vi "TcA02-005_ResizingAttributesCanBeModifiedFasterThanGOOP1.vi"(1 "Input buffer":T3="1", 3 "Invocation info":T2, 5 "error in (no error)":errorcluster, 6 "Add log to result?":bool) -> (16 "Test Data":T1 {"Numeric Measurement" format="%.2f"}, 19 "error out":errorcluster)   [LabVIEW 2020]
doc: "Test case template."
uses:
  Shared/Support_InputBuffer.ctl
  Shared/Support_InvocationInfo.ctl
  Shared/Support_TestData.ctl
  Shared/Support_ResultType.ctl
  TestClasses/G#SubClass1_class/G#SubClass1.lvclass
  TestClasses/G#BaseClass1_class/G#BaseClass1.lvclass
  <vilib>/addons/_AddQ/G#Object/G#Object.lvclass
panel:
  in  "Test name":string="TcA02-005 Resizing attributes can be modified faster than GOOP1"
  out "Test result":bool
  out "Result":string
  # "Verify that object attributes are modified faster\nthan GOOP1 for an attribute that resizes."
  # "Sub test case"
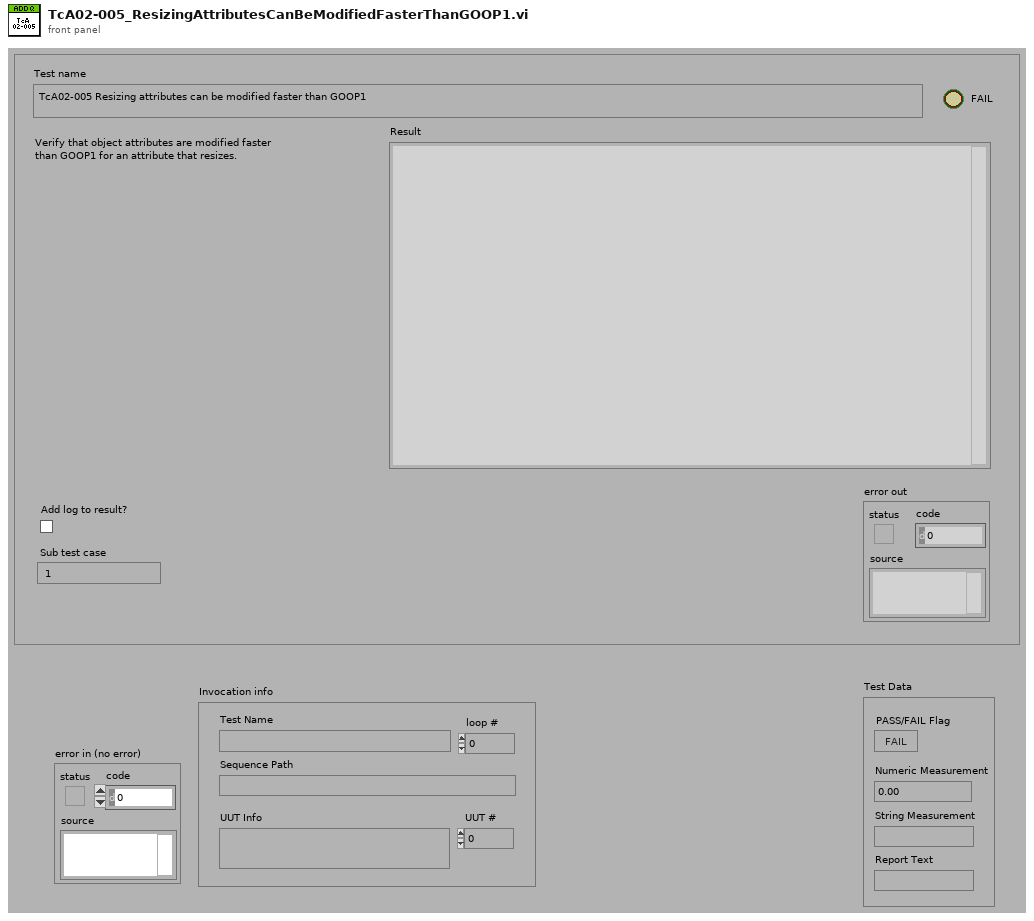
[diagram p1: front panel]
types:
  T1 = typedef "Support_TestData.ctl" = cluster{"PASS/FAIL Flag":bool, "Numeric Measurement":dbl, "String Measurement":string, "Report Text":string}
  T2 = typedef "Support_InvocationInfo.ctl" = cluster{"UUT #":i32, "loop #":i32, "UUT Info":string, "Test Name":string, "Sequence Path":path}
  T3 = typedef "Support_InputBuffer.ctl" = string
  T4 = typedef "Support_ResultType.ctl" = cluster{"Pass":bool, "Comment":string, "MeasurementValue":dbl}
  T5 = typedef "TcOldClass_Object Reference.ctl" = refnum<k1>
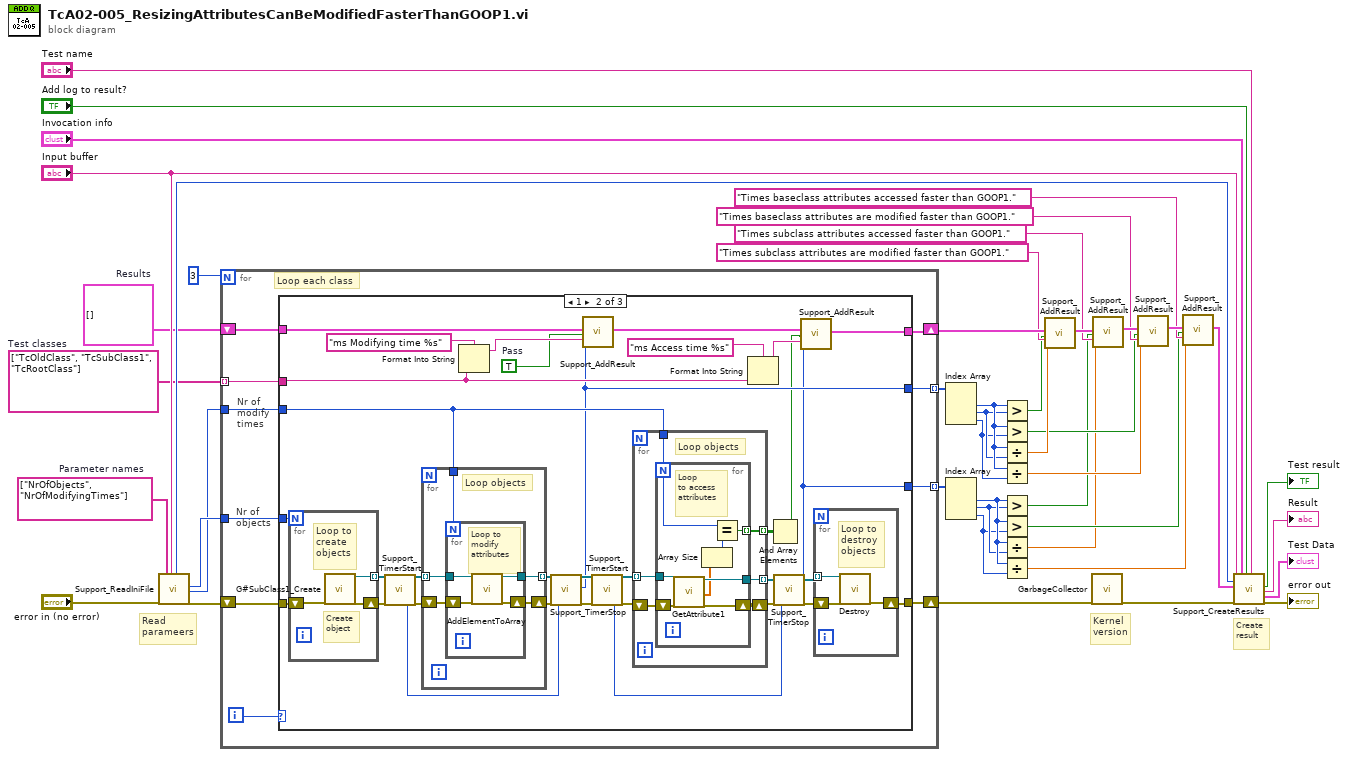
[diagram p0: block diagram]
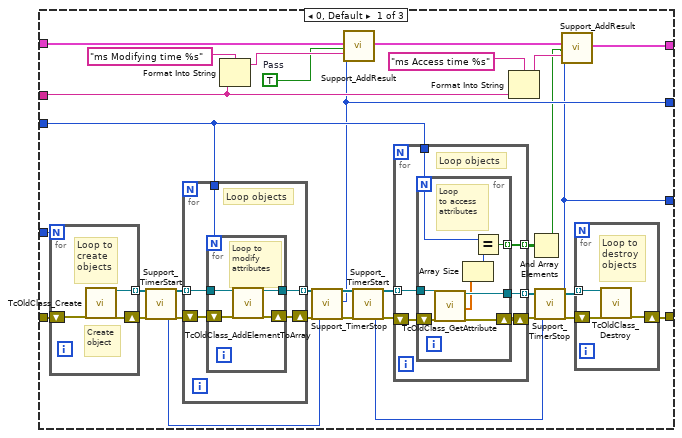
[diagram p2: hidden frame]
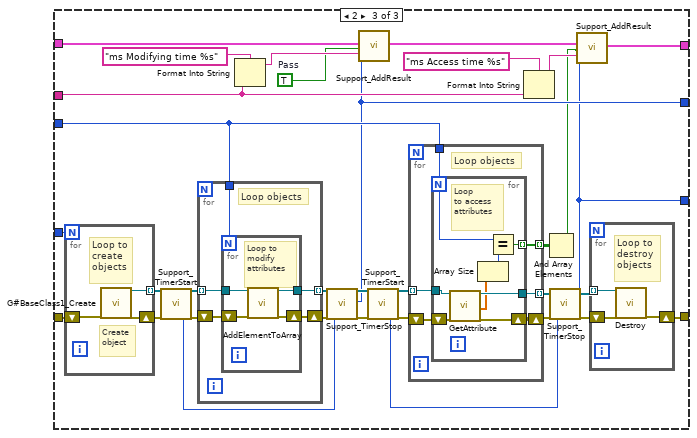
[diagram p3: hidden frame]
diagram:
  w26 = string[] ["TcOldClass", "TcSubClass1", "TcRootClass"]  # Test classes
  w27 = T4[] []  # Results
  w29 = string[] ["NrOfObjects", "NrOfModifyingTimes"]  # Parameter names
  # "Kernel\nversion"
  # "Read\nparameers"
  # "Create\nresult"
  n1 = call "Support_ReadIniFile.vi"("error in (no error)"="error in (no error)", "Parameter names"=w29, "Sub test case"="Input buffer") -> ("Timer start"=w34:u32, "Parameter1 as I32"=w30:i32, "Parameter2 as I32"=w28:i32, "error out"=w31:errorcluster)  [unwired: 9 in, 4 out]
  n2 = for {
    N: 3 -> [_]
    tunnel: w30 -> [w54]
    shift-right: [w52] -> w32
    shift-left: w31 -> [w51]
    tunnel: w28 -> [w50]
    shift-right: [w47] -> w24
    shift-left: w27 -> [w48]
    tunnel: w26 -> [w49] mode=indexing
    tunnel: [w46] -> w20 mode=indexing
    tunnel: [w45] -> w21 mode=indexing
    i -> [w53]
    # "Nr of\nobjects"
    # "Nr of\nmodify\ntimes"
    # "Loop each class"
    n3 = case shown="1" w53 {
      tunnel: w51 -> [w81 w139 w197]
      tunnel: w54 -> [w83 w141 w199]
      tunnel: [w73 w131 w189] -> w52
      tunnel: w50 -> [w70 w128 w186]
      tunnel: w49 -> [w61 w119 w177]
      tunnel: w48 -> [w67 w125 w183]
      tunnel: [w60 w118 w176] -> w47
      tunnel: [w59 w117 w175] -> w46
      tunnel: [w58 w116 w174] -> w45
      frame 0, Default {
        w57 = TRUE  # Pass
        n4 = for {
          N: w83 -> [_]
          shift-right: [w110] -> w80
          shift-left: w81 -> [w111]
          tunnel: [w112] -> w79 mode=indexing
          # "Create\nobject"
          # "Loop to\ncreate\nobjects"
          n5 = call "TcOldClass_Create.vi"("error in (no error)"=w111) -> ("reference"=w112:T5, "error out"=w110:errorcluster)  [unwired: 17 in]
        }
        n6 = call "Support_TimerStart.vi"("error in (no error)"=w80) -> ("Start time"=w82:u32, "error out"=w78:errorcluster)  [unwired: 17 in]
        n7 = for {
          tunnel: w79 -> [w88] mode=indexing
          tunnel: w70 -> [w87]
          tunnel: [w86] -> w71 mode=indexing
          shift-right: [w84] -> w77
          shift-left: w78 -> [w85]
          # "Loop objects"
          n8 = for {
            N: w87 -> [_]
            shift-right: [w91] -> w84
            shift-left: w85 -> [w92]
            tunnel: w88 -> [w90]
            tunnel: [w89] -> w86
            # "Loop to\nmodify\nattributes"
            n9 = call "TcOldClass_AddElementToArray.vi"("reference"=w90, "error in (no error)"=w92) -> ("duplicate reference"=w89:T5, "error out"=w91:errorcluster)  [unwired: 16 in]
          }
        }
        n10 = Format Into String(format string="ms Modifying time %s", w61) -> (resulting string=w65:string)  [unwired: 2 in, 1 out]
        n11 = call "Support_TimerStop.vi"("error in (no error)"=w77, "Start time"=w82) -> ("Time (ms)"=w59:u32, "error out"=w76:errorcluster)  [unwired: 16 in]
        n12 = call "Support_AddResult.vi"("Results in"=w67, "Pass"=w57, "Comment"=w65, "MeasurementValue"=w59) -> ("Results out"=w64:T4[])  [unwired: 15 in]
        n13 = call "Support_TimerStart.vi"("error in (no error)"=w76) -> ("Start time"=w68:u32, "error out"=w75:errorcluster)  [unwired: 17 in]
        n14 = for {
          shift-right: [w97] -> w74
          shift-left: w75 -> [w98]
          tunnel: w71 -> [w96] mode=indexing
          tunnel: w70 -> [w95]
          tunnel: [w94] -> w69 mode=indexing
          tunnel: [w93] -> w55 mode=indexing
          # "Loop objects"
          n15 = for {
            N: w95 -> [w100]
            shift-right: [w105] -> w97
            shift-left: w98 -> [w106]
            tunnel: w96 -> [w104]
            tunnel: [w103] -> w94
            tunnel: [w99] -> w93 mode=indexing
            # "Loop\nto access\nattributes"
            n16 = call "TcOldClass_GetAttribute.vi"("reference"=w104, "error in (no error)"=w106) -> ("duplicate reference"=w103:T5, "tcRootArray"=w102:dbl[], "error out"=w105:errorcluster)  [unwired: 13 in, 2 out]
            n17 = Array Size(array=w102) -> (size(s)=w101:i32)
            n18 = Equal?(x=w100, y=w101) -> (x = y?=w99:bool)
          }
        }
        n19 = Format Into String(format string="ms Access time %s", w61) -> (resulting string=w63:string)  [unwired: 2 in, 1 out]
        n20 = And Array Elements(Boolean array=w55) -> (logical AND=w56:bool)
        n21 = call "Support_TimerStop.vi"("error in (no error)"=w74, "Start time"=w68) -> ("Time (ms)"=w58:u32, "error out"=w72:errorcluster)  [unwired: 16 in]
        n22 = call "Support_AddResult.vi"("Results in"=w64, "Pass"=w56, "Comment"=w63, "MeasurementValue"=w58) -> ("Results out"=w60:T4[])  [unwired: 15 in]
        n23 = for {
          tunnel: w69 -> [w109] mode=indexing
          shift-right: [w107] -> w73
          shift-left: w72 -> [w108]
          # "Loop to \ndestroy\nobjects"
          n24 = call "TcOldClass_Destroy.vi"("reference"=w109, "error in (no error)"=w108) -> ("error out"=w107:errorcluster)  [unwired: 17 in]
        }
      }
      frame 1 {
        w115 = TRUE  # Pass
        n25 = for {
          N: w141 -> [_]
          shift-right: [w169] -> w138
          shift-left: w139 -> [w170]
          tunnel: [w168] -> w137 mode=indexing
          # "Create\nobject"
          # "Loop to\ncreate\nobjects"
          n26 = call "G#SubClass1_Create.vi"("error in (no error)"=w170) -> ("reference out"=w168:refnum<class "G#SubClass1.lvclass">, "error out"=w169:errorcluster)  [unwired: 16 in, 1 out]
        }
        n27 = call "Support_TimerStart.vi"("error in (no error)"=w138) -> ("Start time"=w140:u32, "error out"=w136:errorcluster)  [unwired: 17 in]
        n28 = for {
          tunnel: w137 -> [w146] mode=indexing
          tunnel: w128 -> [w145]
          tunnel: [w144] -> w129 mode=indexing
          shift-right: [w142] -> w135
          shift-left: w136 -> [w143]
          # "Loop objects"
          n29 = for {
            N: w145 -> [_]
            shift-right: [w149] -> w142
            shift-left: w143 -> [w150]
            tunnel: w146 -> [w148]
            tunnel: [w147] -> w144
            # "Loop to\nmodify\nattributes"
            n30 = call-dynamic "AddElementToArray.vi"("reference in"=w148, "error in (no error)"=w150) -> ("reference out"=w147:refnum<class "G#SubClass1.lvclass">, "error out"=w149:errorcluster)  [unwired: 16 in]
          }
        }
        n31 = Format Into String(format string="ms Modifying time %s", w119) -> (resulting string=w123:string)  [unwired: 2 in, 1 out]
        n32 = call "Support_TimerStop.vi"("error in (no error)"=w135, "Start time"=w140) -> ("Time (ms)"=w117:u32, "error out"=w134:errorcluster)  [unwired: 16 in]
        n33 = call "Support_AddResult.vi"("Results in"=w125, "Pass"=w115, "Comment"=w123, "MeasurementValue"=w117) -> ("Results out"=w122:T4[])  [unwired: 15 in]
        n34 = call "Support_TimerStart.vi"("error in (no error)"=w134) -> ("Start time"=w126:u32, "error out"=w133:errorcluster)  [unwired: 17 in]
        n35 = for {
          shift-right: [w155] -> w132
          shift-left: w133 -> [w156]
          tunnel: w129 -> [w154] mode=indexing
          tunnel: w128 -> [w153]
          tunnel: [w152] -> w127 mode=indexing
          tunnel: [w151] -> w113 mode=indexing
          # "Loop objects"
          n36 = for {
            N: w153 -> [w158]
            shift-right: [w163] -> w155
            shift-left: w156 -> [w164]
            tunnel: w154 -> [w162]
            tunnel: [w161] -> w152
            tunnel: [w157] -> w151 mode=indexing
            # "Loop\nto access\nattributes"
            n37 = call-dynamic "GetAttribute1.vi"("reference in"=w162, "error in (no error)"=w164) -> ("reference out"=w161:refnum<class "G#SubClass1.lvclass">, "Base class.Array"=w160:dbl[], "error out"=w163:errorcluster)  [unwired: 13 in, 2 out]
            n38 = Array Size(array=w160) -> (size(s)=w159:i32)
            n39 = Equal?(x=w158, y=w159) -> (x = y?=w157:bool)
          }
        }
        n40 = Format Into String(format string="ms Access time %s", w119) -> (resulting string=w121:string)  [unwired: 2 in, 1 out]
        n41 = And Array Elements(Boolean array=w113) -> (logical AND=w114:bool)
        n42 = call "Support_TimerStop.vi"("error in (no error)"=w132, "Start time"=w126) -> ("Time (ms)"=w116:u32, "error out"=w130:errorcluster)  [unwired: 16 in]
        n43 = call "Support_AddResult.vi"("Results in"=w122, "Pass"=w114, "Comment"=w121, "MeasurementValue"=w116) -> ("Results out"=w118:T4[])  [unwired: 15 in]
        n44 = for {
          tunnel: w127 -> [w167] mode=indexing
          shift-right: [w165] -> w131
          shift-left: w130 -> [w166]
          # "Loop to \ndestroy\nobjects"
          n45 = call-dynamic "Destroy.vi"("reference in"=w167, "error in (no error)"=w166) -> ("error out"=w165:errorcluster)  [unwired: 16 in, 1 out]
        }
      }
      frame 2 {
        w173 = TRUE  # Pass
        n46 = for {
          N: w199 -> [_]
          shift-right: [w227] -> w196
          shift-left: w197 -> [w228]
          tunnel: [w226] -> w195 mode=indexing
          # "Create\nobject"
          # "Loop to\ncreate\nobjects"
          n47 = call "G#BaseClass1_Create.vi"("error in (no error)"=w228) -> ("reference out"=w226:refnum<class "G#BaseClass1.lvclass">, "error out"=w227:errorcluster)  [unwired: 16 in, 1 out]
        }
        n48 = call "Support_TimerStart.vi"("error in (no error)"=w196) -> ("Start time"=w198:u32, "error out"=w194:errorcluster)  [unwired: 17 in]
        n49 = for {
          tunnel: w195 -> [w204] mode=indexing
          tunnel: w186 -> [w203]
          tunnel: [w202] -> w187 mode=indexing
          shift-right: [w200] -> w193
          shift-left: w194 -> [w201]
          # "Loop objects"
          n50 = for {
            N: w203 -> [_]
            shift-right: [w207] -> w200
            shift-left: w201 -> [w208]
            tunnel: w204 -> [w206]
            tunnel: [w205] -> w202
            # "Loop to\nmodify\nattributes"
            n51 = call-dynamic "AddElementToArray.vi"("reference in"=w206, "error in (no error)"=w208) -> ("reference out"=w205:refnum<class "G#BaseClass1.lvclass">, "error out"=w207:errorcluster)  [unwired: 16 in]
          }
        }
        n52 = Format Into String(format string="ms Modifying time %s", w177) -> (resulting string=w181:string)  [unwired: 2 in, 1 out]
        n53 = call "Support_TimerStop.vi"("error in (no error)"=w193, "Start time"=w198) -> ("Time (ms)"=w175:u32, "error out"=w192:errorcluster)  [unwired: 16 in]
        n54 = call "Support_AddResult.vi"("Results in"=w183, "Pass"=w173, "Comment"=w181, "MeasurementValue"=w175) -> ("Results out"=w180:T4[])  [unwired: 15 in]
        n55 = call "Support_TimerStart.vi"("error in (no error)"=w192) -> ("Start time"=w184:u32, "error out"=w191:errorcluster)  [unwired: 17 in]
        n56 = for {
          shift-right: [w213] -> w190
          shift-left: w191 -> [w214]
          tunnel: w187 -> [w212] mode=indexing
          tunnel: w186 -> [w211]
          tunnel: [w210] -> w185 mode=indexing
          tunnel: [w209] -> w171 mode=indexing
          # "Loop objects"
          n57 = for {
            N: w211 -> [w217]
            shift-right: [w221] -> w213
            shift-left: w214 -> [w222]
            tunnel: w212 -> [w215]
            tunnel: [w220] -> w210
            tunnel: [w216] -> w209 mode=indexing
            # "Loop\nto access\nattributes"
            n58 = call-dynamic "GetAttribute.vi"("reference in"=w215, "error in (no error)"=w222) -> ("reference out"=w220:refnum<class "G#BaseClass1.lvclass">, "Array"=w219:dbl[], "error out"=w221:errorcluster)  [unwired: 14 in, 1 out]
            n59 = Array Size(array=w219) -> (size(s)=w218:i32)
            n60 = Equal?(x=w217, y=w218) -> (x = y?=w216:bool)
          }
        }
        n61 = Format Into String(format string="ms Access time %s", w177) -> (resulting string=w179:string)  [unwired: 2 in, 1 out]
        n62 = And Array Elements(Boolean array=w171) -> (logical AND=w172:bool)
        n63 = call "Support_TimerStop.vi"("error in (no error)"=w190, "Start time"=w184) -> ("Time (ms)"=w174:u32, "error out"=w188:errorcluster)  [unwired: 16 in]
        n64 = call "Support_AddResult.vi"("Results in"=w180, "Pass"=w172, "Comment"=w179, "MeasurementValue"=w174) -> ("Results out"=w176:T4[])  [unwired: 15 in]
        n65 = for {
          tunnel: w185 -> [w225] mode=indexing
          shift-right: [w223] -> w189
          shift-left: w188 -> [w224]
          # "Loop to \ndestroy\nobjects"
          n66 = call-dynamic "Destroy.vi"("reference in"=w225, "error in (no error)"=w224) -> ("error out"=w223:errorcluster)  [unwired: 16 in, 1 out]
        }
      }
    }
  }
  n67 = Index Array(array=w20) -> (element #1=w14:u32, element #2=w12:u32, element #3=w11:u32)  [unwired: 3 in]
  n68 = Index Array(array=w21) -> (element #1=w13:u32, element #2=w10:u32, element #3=w9:u32)  [unwired: 3 in]
  n69 = Greater?(x=w14, y=w12) -> (0:w8:bool)
  n70 = Greater?(x=w14, y=w11) -> (0:w6:bool)
  n71 = Divide(x=w14, y=w12) -> (x/y=w7:dbl)
  n72 = Divide(x=w14, y=w11) -> (x/y=w5:dbl)
  n73 = Greater?(x=w13, y=w10) -> (0:w4:bool)
  n74 = Greater?(x=w13, y=w9) -> (0:w3:bool)
  n75 = Divide(x=w13, y=w10) -> (x/y=w2:dbl)
  n76 = Divide(x=w13, y=w9) -> (x/y=w1:dbl)
  n77 = call "Support_AddResult.vi"("Results in"=w24, "Pass"=w8, "Comment"="Times subclass attributes are modified faster than GOOP1.", "MeasurementValue"=w7) -> ("Results out"=w25:T4[])  [unwired: 15 in]
  n78 = call <vilib>:"GarbageCollector.vi"("error in (no error)"=w32) -> ("error out"=w36:errorcluster)  [unwired: 16 in, 2 out]
  n79 = call "Support_AddResult.vi"("Results in"=w25, "Pass"=w4, "Comment"="Times subclass attributes accessed faster than GOOP1.", "MeasurementValue"=w2) -> ("Results out"=w19:T4[])  [unwired: 15 in]
  n80 = call "Support_AddResult.vi"("Results in"=w19, "Pass"=w6, "Comment"="Times baseclass attributes are modified faster than GOOP1.", "MeasurementValue"=w5) -> ("Results out"=w17:T4[])  [unwired: 15 in]
  n81 = call "Support_AddResult.vi"("Results in"=w17, "Pass"=w3, "Comment"="Times baseclass attributes accessed faster than GOOP1.", "MeasurementValue"=w1) -> ("Results out"=w18:T4[])  [unwired: 15 in]
  n82 = call "Support_CreateResults.vi"("Sub test case"="Input buffer", "Timer start"=w34, "Results"=w18, "error in (no error)"=w36, "Invocation info"="Invocation info", "Add log to result?"="Add log to result?", "Test name"="Test name") -> ("Pass/fail flag"=→"Test result":bool, "Result"=→"Result":string, "Test Data"=→"Test Data":T1, "error out"=→"error out":errorcluster)  [unwired: 9 in]
